vi "GlobalReverseFlag.vi"() -> ()   [LabVIEW 2010]
panel:
  out "Reverse Active":bool
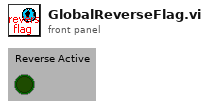
[diagram p1: front panel]
diagram:
